vi "Write OS Endian.vi"(8 "error in (no error)":errorcluster, 10 "Endian":T1, 11 "pcap_Parse_Build_CIF in":refnum<class "pcap_Parse_Build_CIF.lvclass">) -> (0 "error out":errorcluster, 3 "pcap_Parse_Build_CIF out":refnum<class "pcap_Parse_Build_CIF.lvclass">)   [LabVIEW 2021, in "pcap_Parse_Build_CIF.lvclass"]
doc: "This is automatically detected and set when the PCP class is initialized. It is an advanced feature to override this setting."
uses:
  pcap_Parse_Build_CIF.lvclass
  pcap_Parse_Build_CIF.lvclass/pcap_Parse_Build_CIF.ctl
  <vilib>/CIF Foundation/CIF Utilities/DataTypes/Typedef/Endian.ctl
  <vilib>/CIF Foundation/CIF Utilities/DataTypes/DataTypes_CIF_U.lvlib
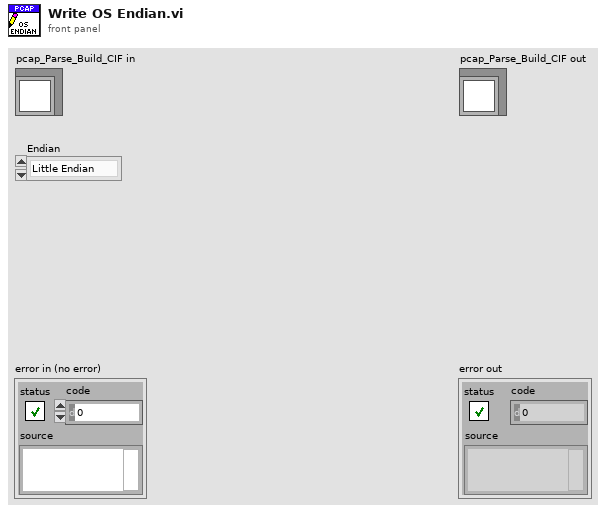
[diagram p1: front panel]
types:
  T1 = typedef "DataTypes_CIF_U.lvlib/Endian.ctl" = enum16{"Little Endian", "Big Endian"}
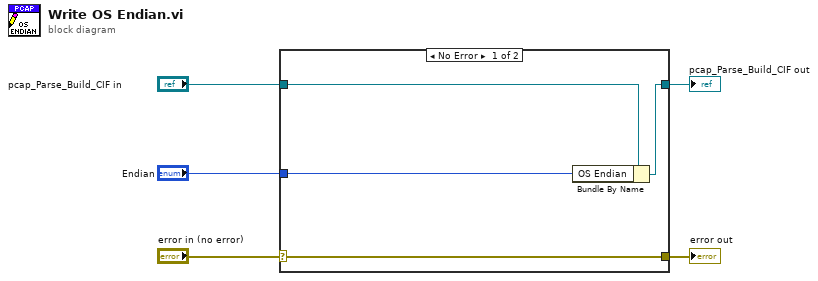
[diagram p0: block diagram]
diagram:
  n1 = case shown="No Error" "error in (no error)" {
    selector: "error in (no error)" -> [w9 w10]
    tunnel: [w9 w10] -> w4
    tunnel: [w7 w11] -> w2
    tunnel: "pcap_Parse_Build_CIF in" -> [w8 w11]
    tunnel: "Endian" -> [w6 _]
    frame No Error {
      n2 = Bundle By Name(cluster=w8, "OS Endian"=w6) -> (w7:refnum<class "pcap_Parse_Build_CIF.lvclass">)
    }
    frame Error {
    }
  }
  "error out" <- w4
  "pcap_Parse_Build_CIF out" <- w2
